vi "Arrange all data in column (for saving).vi"(7 "Time (s)":dbl, 8 "ZVL":T2, 9 "Lock-in Amplifier":T1, 10 "Lakeshore":T3, 11 "Magnetic field":T4) -> (3 "Result string (for saving)":string)   [LabVIEW 2019]
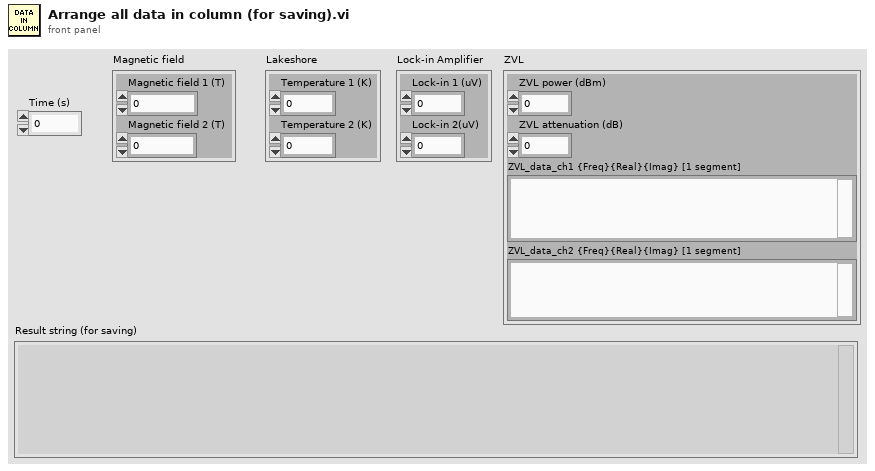
[diagram p1: front panel]
types:
  T1 = cluster{"Lock-in 1 (uV)":dbl, "Lock-in 2(uV)":dbl}
  T2 = cluster{"ZVL power (dBm)":dbl, "ZVL attenuation (dB)":dbl, "ZVL_data_ch1 {Freq}{Real}{Imag} [1 segment]":string, "ZVL_data_ch2 {Freq}{Real}{Imag} [1 segment]":string}
  T3 = cluster{"Temperature 1 (K)":dbl, "Temperature 2 (K)":dbl}
  T4 = cluster{"Magnetic field 1 (T)":dbl, "Magnetic field 2 (T)":dbl}
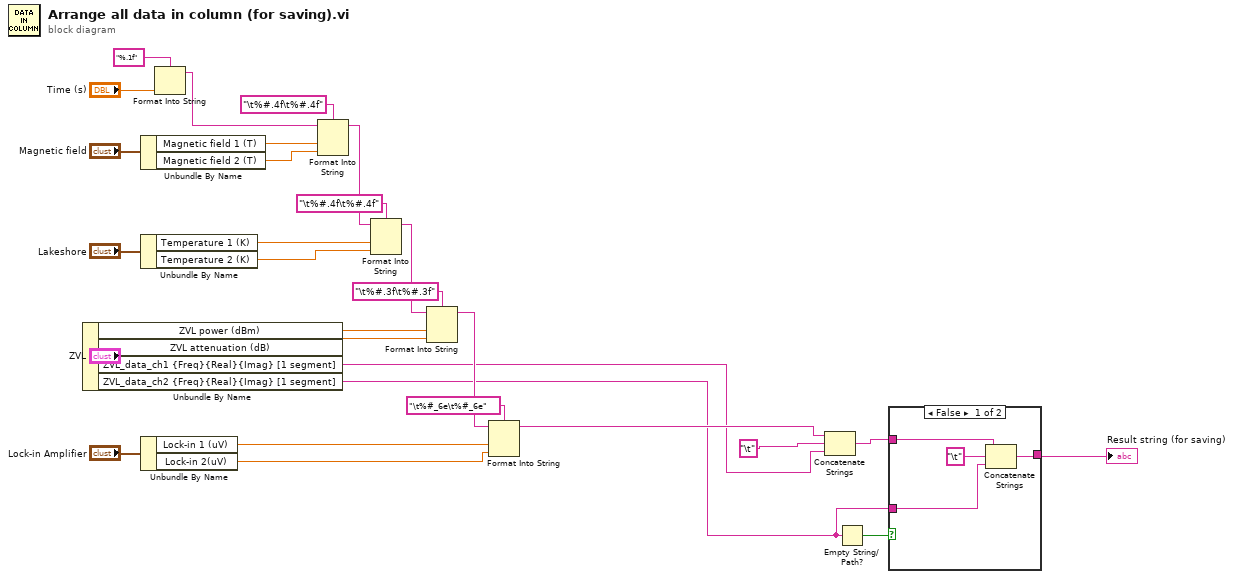
[diagram p0: block diagram]
diagram:
  n1 = Unbundle By Name("ZVL") -> ("ZVL power (dBm)"=w10:dbl, "ZVL attenuation (dB)"=w9:dbl, "ZVL_data_ch1 {Freq}{Real}{Imag} [1 segment]"=w2:string, "ZVL_data_ch2 {Freq}{Real}{Imag} [1 segment]"=w1:string)
  n2 = Unbundle By Name("Magnetic field") -> ("Magnetic field 1 (T)"=w17:dbl, "Magnetic field 2 (T)"=w16:dbl)
  n3 = Unbundle By Name("Lakeshore") -> ("Temperature 1 (K)"=w14:dbl, "Temperature 2 (K)"=w13:dbl)
  n4 = Unbundle By Name("Lock-in Amplifier") -> ("Lock-in 1 (uV)"=w5:dbl, "Lock-in 2(uV)"=w4:dbl)
  n5 = Format Into String(format string="%.1f" ("Cmd string"), "Time (s)") -> (resulting string=w19:string)  [unwired: 2 in, 1 out]
  n6 = Format Into String(format string="\t%#.4f\t%#.4f" ("Cmd string"), initial string=w19, w17, w16) -> (resulting string=w12:string)  [unwired: 1 in, 1 out]
  n7 = Format Into String(format string="\t%#.4f\t%#.4f" ("Cmd string"), initial string=w12, w14, w13) -> (resulting string=w8:string)  [unwired: 1 in, 1 out]
  n8 = Format Into String(format string="\t%#.3f\t%#.3f" ("Cmd string"), initial string=w8, w10, w9) -> (resulting string=w6:string)  [unwired: 1 in, 1 out]
  n9 = Format Into String(format string="\t%#_6e\t%#_6e" ("Cmd string"), initial string=w6, w5, w4) -> (resulting string=w3:string)  [unwired: 1 in, 1 out]
  n10 = Concatenate Strings(w3, "\t" ("string"), w2) -> (w25:string)
  n11 = Empty String/Path?(string/path=w1) -> (empty?=w26:bool)
  n12 = case shown="False" w26 {
    tunnel: w25 -> [w33 w34]
    tunnel: [w30 w34] -> w24
    tunnel: w1 -> [w32 _]
    frame False {
      n13 = Concatenate Strings(w33, "\t" ("string"), w32) -> (w30:string)
    }
    frame True {
    }
  }
  "Result string (for saving)" <- w24
